vi "Get Available Pointers by Type.vi"(5 "Test Executive Builder Data Type Handler in":refnum<class "Test Executive Builder Data Type Handler.lvclass">, 7 "ID":string, 8 "error in (no error)":errorcluster, 9 "Type":variant, 11 "Test Executive Ref":refnum<data-value>) -> (0 "error out":errorcluster, 1 "Names":string[](array[string]), 2 "IDs":string[](array[string]), 3 "Test Executive Ref out":refnum<data-value>)   [LabVIEW 2017, in "Test Executive Builder Data Type Handler.lvclass"]
uses:
  Test Executive Builder Data Type Handler.lvclass
  <vilib>/gpm_packages/@cs/test-executive/Source/Test Executive/ITestExecutive/ITest Executive.lvclass
  Test Executive Builder Dialogs/LimitType/Numeric Limit.ctl
  d747f5b8-90c1-47a6-a349-03b9408ce2fe.vi
  db82b9ad-c723-4df7-8ad0-3d3813c8c626.vi
  e8722132-6a20-4652-a547-1b4d262eb7e3.vi
  14b15206-fe2b-411d-8f8c-447e995964d5.vi
  7c85d718-3dcd-40bb-a5d0-f70cd0e004ea.vi
  <vilib>/Utility/error.llb/Clear Errors.vi
  <vilib>/Utility/Data Type/NI_Data Type.lvlib
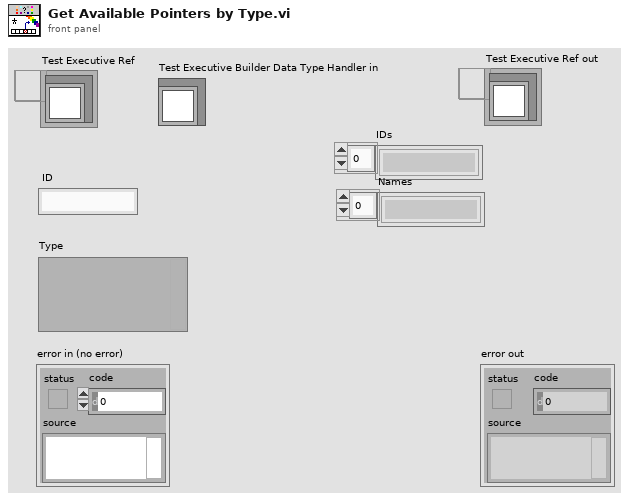
[diagram p1: front panel]
types:
  T1 = typedef "NI_Data Type.lvlib/Data Type.ctl" = enum8{"Invalid Type", "Void", "I8", "I16", "I32", "I64", "U8", "U16", "U32", "U64", "Single Float", "Double Float", "Extended Float", "Single Complex", "Double Complex", "Extended Complex", "Enum U8", "Enum U16", "Enum U32", "Enum U64", "Single Float With Unit", "Double Float With Unit", "Extended Float With Unit", "Single Complex with Unit", "Double Complex with Unit", "Extended Complex with Unit", "Boolean", "String", "Path", "Picture", "Tag", "Array", "Cluster", "Variant", "LV Variant", "Waveform", "Timestamp", "Digital Waveform", "Digital Data", "ExpressData", "Refnum", "External Data", "VI", "Poly VI", "LabVIEW Class Instance", "Fixed Point"}
  T2 = typedef "Numeric Limit.ctl" = cluster{"High Limit":dbl, "Low Limit":dbl, "Check Item":string, "Assertion HIGH":u16, "Assertion LOW":u16}
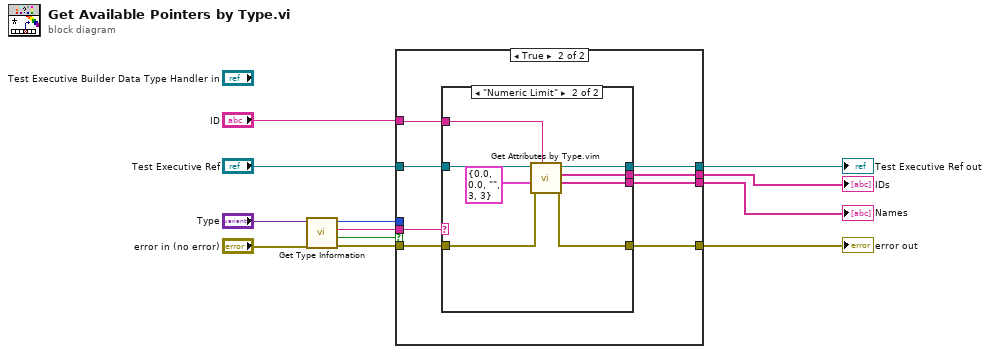
[diagram p0: block diagram]
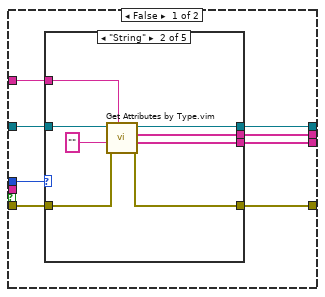
[diagram p2: hidden frame]
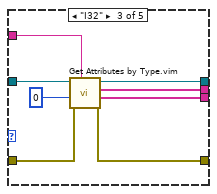
[diagram p4: hidden frame]
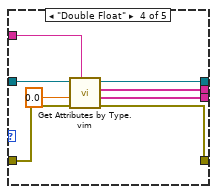
[diagram p5: hidden frame]
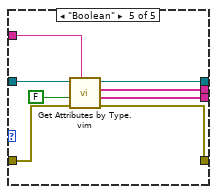
[diagram p6: hidden frame]
diagram:
  n1 = call <vilib>:"Get Type Information.vi"("error in (no error)"="error in (no error)", "Variant"="Type") -> ("error out"=w6:errorcluster, "Type Definition"=w2:bool, "Name"=w1:string, "Type"=w3:T1)  [unwired: 5 in, 1 out]
  n2 = case shown="True" w2 {
    tunnel: "Test Executive Ref" -> [w20 w61]
    tunnel: [w19 w60] -> w11
    tunnel: "ID" -> [w18 w62]
    tunnel: [w17 w57] -> w8
    tunnel: [w16 w56] -> w7
    tunnel: w6 -> [w15 w59]
    tunnel: [w14 w58] -> w4
    tunnel: w3 -> [w13 _]
    tunnel: w1 -> [_ w55]
    frame False {
      n3 = case shown="\"String\"" w13 {
        tunnel: w20 -> [w22 w30 w38 w46 w54]
        tunnel: [w22 w29 w37 w45 w53] -> w19
        tunnel: w18 -> [_ w28 w36 w44 w52]
        tunnel: [_ w27 w35 w43 w51] -> w17
        tunnel: [_ w26 w34 w42 w50] -> w16
        tunnel: w15 -> [w21 w25 w33 w41 w49]
        tunnel: [w21 w24 w32 w40 w48] -> w14
        frame Default {
        }
        frame "String" {
          n4 = call "Get Attributes by Type.vim"("ID"=w28, "error in (no error)"=w25, "Type"="", "Test Executive Ref"=w30) -> ("error out"=w24:errorcluster, "Names"=w26:string[], "IDs"=w27:string[], "Test Executive Ref out"=w29:refnum<data-value>)  [unwired: 3 in, 1 out]
        }
        frame "I32" {
          n5 = call "Get Attributes by Type.vim"("ID"=w36, "error in (no error)"=w33, "Type"=0, "Test Executive Ref"=w38) -> ("error out"=w32:errorcluster, "Names"=w34:string[], "IDs"=w35:string[], "Test Executive Ref out"=w37:refnum<data-value>)  [unwired: 3 in, 1 out]
        }
        frame "Double Float" {
          n6 = call "Get Attributes by Type.vim"("ID"=w44, "error in (no error)"=w41, "Type"=0.0, "Test Executive Ref"=w46) -> ("error out"=w40:errorcluster, "Names"=w42:string[], "IDs"=w43:string[], "Test Executive Ref out"=w45:refnum<data-value>)  [unwired: 3 in, 1 out]
        }
        frame "Boolean" {
          n7 = call "Get Attributes by Type.vim"("ID"=w52, "error in (no error)"=w49, "Type"=FALSE, "Test Executive Ref"=w54) -> ("error out"=w48:errorcluster, "Names"=w50:string[], "IDs"=w51:string[], "Test Executive Ref out"=w53:refnum<data-value>)  [unwired: 3 in, 1 out]
        }
      }
    }
    frame True {
      n8 = case shown="\"Numeric Limit\"" w55 {
        tunnel: w62 -> [_ w72]
        tunnel: w61 -> [w63 w71]
        tunnel: [w63 w70] -> w60
        tunnel: w59 -> [w64 w69]
        tunnel: [w64 w68] -> w58
        tunnel: [_ w67] -> w57
        tunnel: [_ w66] -> w56
        frame "False", Default {
        }
        frame "Numeric Limit" {
          n9 = call "Get Attributes by Type.vim"("ID"=w72, "error in (no error)"=w69, "Type"=T2 {"High Limit"=0.0, "Low Limit"=0.0, "Check Item"="", "Assertion HIGH"=3, "Assertion LOW"=3} ("Numeric Limit"), "Test Executive Ref"=w71) -> ("error out"=w68:errorcluster, "Names"=w66:string[], "IDs"=w67:string[], "Test Executive Ref out"=w70:refnum<data-value>)  [unwired: 3 in, 1 out]
        }
      }
    }
  }
  "error out" <- w4
  "Test Executive Ref out" <- w11
  "IDs" <- w8
  "Names" <- w7
